vi "detectedCameras.vi"(7 "action":T2, 8 "error in (no error)":errorcluster, 11 "Discovered Cameras":T1[](array[typedef])) -> (0 "error out":errorcluster, 3 "Discovered Cameras":T1[](array[typedef]))   [LabVIEW 2017, in "VisionWebServiceData.lvlib"]
uses:
  VisionWebServiceData.lvlib
  action.ctl
  <vilib>/addons/InsightCM/Devices/Shared/Ir/IrManageCameras/controls/camera.ctl
  <vilib>/addons/InsightCM/Devices/Shared/Ir/IrManageCameras/IrManageCameras.lvlib
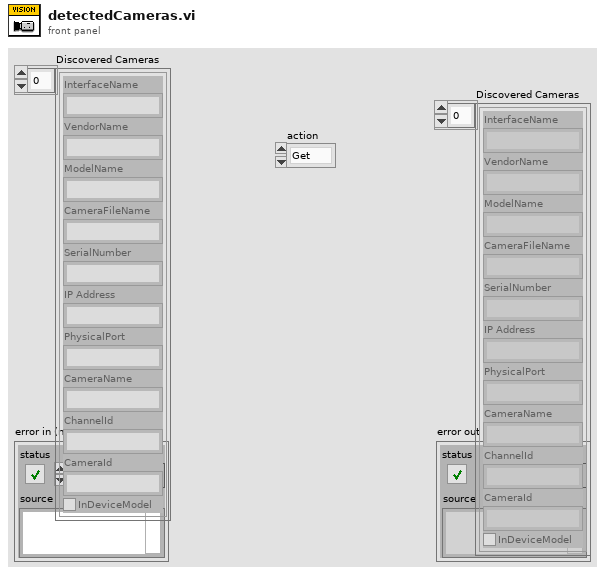
[diagram p1: front panel]
types:
  T1 = typedef "IrManageCameras.lvlib/camera.ctl" = cluster{"InterfaceName":string, "VendorName":string, "ModelName":string, "CameraFileName":string, "SerialNumber":string, "IP Address":string, "PhysicalPort":string, "CameraName":string, "ChannelId":string, "CameraId":string, "InDeviceModel":bool}
  T2 = typedef "VisionWebServiceData.lvlib/action.ctl" = enum16{"Get", "Set"}
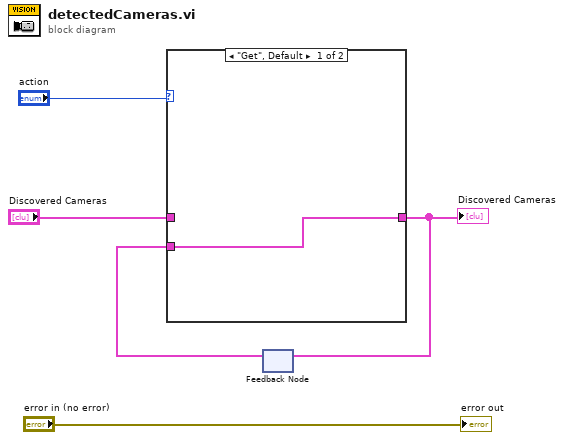
[diagram p0: block diagram]
diagram:
  n1 = feedback #1() -> (w2:T1[])  [unwired: 1 in]
  n2 = case shown="\"Get\", Default" "action" {
    tunnel: "Discovered Cameras" -> [_ w7]
    tunnel: [w6 w7] -> w3
    tunnel: w2 -> [w6 _]
    frame "Get", Default {
    }
    frame "Set" {
    }
  }
  "Discovered Cameras" <- w3
  n3 = feedback-in #1(w3) -> ()
  "error out" <- "error in (no error)"
